vi "Open Connection DriverConnect.vi"(5 "error in (no error)":errorcluster, 6 "Password (\"\")":string, 7 "Username (\"\")":string, 8 "ODBC Database (\"\")":path) -> (0 "error out":errorcluster, 3 "Connection Refnum":T1)   [LabVIEW 2011]
doc: "Réalise l'ensemble des étapes nécéssaires à la mise en place de la connection avec la base de données. Etablit le cas échéant l'utilisation des transactions."
uses:
  SQL Controls/Connection Refnum.ctl
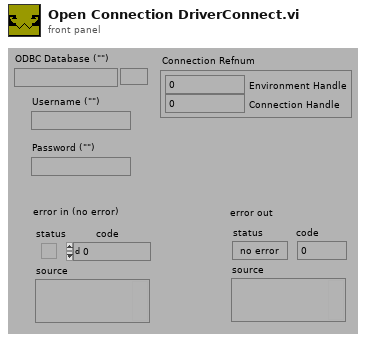
[diagram p1: front panel]
types:
  T1 = typedef "Connection Refnum.ctl" = cluster{"Environment Handle":i32, "Connection Handle":i32}
  T2 = cluster{"Environment Handle":i32, "Connection Handle":i32}
  T3 = enum16{"NOPE", "SQL_HANDLE_ENV", "SQL_HANDLE_DBC", "SQL_HANDLE_STMT", "SQL_HANDLE_DESC"}
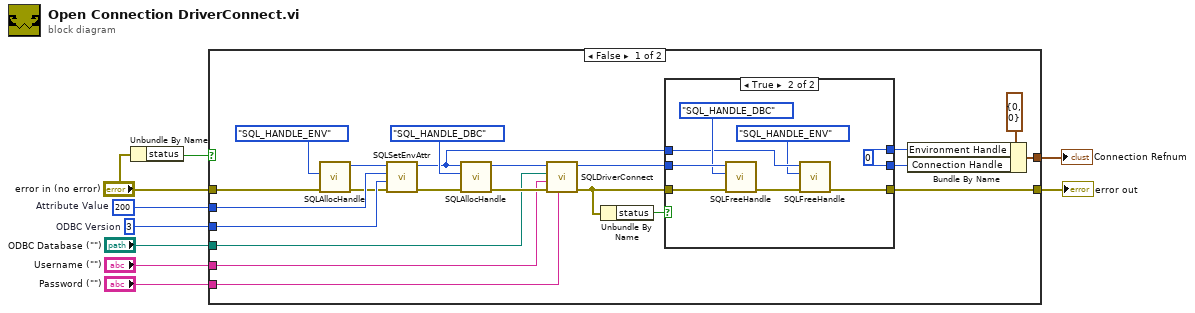
[diagram p0: block diagram]
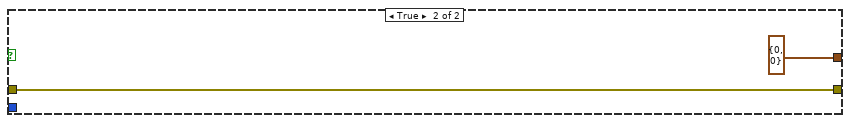
[diagram p3: hidden frame]
diagram:
  w5 = u32 3  # ODBC Version
  w6 = 200  # Attribute Value
  n1 = Unbundle By Name("error in (no error)") -> ("status"=w1:bool)
  n2 = case shown="False" w1 {
    tunnel: "Username (\"\")" -> [w12 _]
    tunnel: "ODBC Database (\"\")" -> [w10 _]
    tunnel: "Password (\"\")" -> [w11 _]
    tunnel: w6 -> [w28 _]
    tunnel: w5 -> [w27 _]
    tunnel: [w24 T2 {"Environment Handle"=0, "Connection Handle"=0} ("Connection Refnum")] -> w4
    tunnel: [w18 w44] -> w3
    tunnel: "error in (no error)" -> [w17 w44]
    frame False {
      n3 = call "SQLAllocHandle.vi"("error in (no error)"=w17, "HandleType"=T3."SQL_HANDLE_ENV") -> ("error out"=w21:errorcluster, "OutputHandle"=w26:i32)  [unwired: 1 in, 3 out]
      n4 = call "SQLSetEnvAttr.vi"("error in (no error)"=w21, "AttributeValue"=w27, "AttributePosition"=w28, "InputHandle"=w26) -> ("error out"=w20:errorcluster, "OutputHandle"=w29:i32)  [unwired: 2 out]
      n5 = call "SQLAllocHandle.vi"("error in (no error)"=w20, "HandleType"=T3."SQL_HANDLE_DBC", "InputHandle"=w29) -> ("error out"=w14:errorcluster, "OutputHandle"=w16:i32)  [unwired: 3 out]
      n6 = call "SQLDriverConnect.vi"("Password"=w11, "error in (no error)"=w14, "UserName"=w12, "Database Path (empty)"=w10, "InputHandle"=w16) -> ("error out"=w13:errorcluster, "OutputHandle"=w15:i32)  [unwired: 2 out]
      n7 = Unbundle By Name(w13) -> ("status"=w19:bool)
      n8 = case shown="True" w19 {
        tunnel: w15 -> [w33 w42]
        tunnel: w29 -> [w34 w38]
        tunnel: [w34 w41] -> w23
        tunnel: [w33 w41] -> w22
        tunnel: [w32 w36] -> w18
        tunnel: w13 -> [w32 w35]
        frame False {
        }
        frame True {
          w41 = 0 ("OutputHandle")
          n9 = call "SQLFreeHandle.vi"("error in (no error)"=w35, "HandleType"=T3."SQL_HANDLE_DBC", "InputHandle"=w42) -> ("error out"=w39:errorcluster)  [unwired: 4 out]
          n10 = call "SQLFreeHandle.vi"("error in (no error)"=w39, "HandleType"=T3."SQL_HANDLE_ENV", "InputHandle"=w38) -> ("error out"=w36:errorcluster)  [unwired: 4 out]
        }
      }
      n11 = Bundle By Name(cluster=T2 {"Environment Handle"=0, "Connection Handle"=0} ("Connection Refnum"), "Environment Handle"=w23, "Connection Handle"=w22) -> (w24:T2)
    }
    frame True {
    }
  }
  "Connection Refnum" <- w4
  "error out" <- w3
